vi "Test Ultrasonic Sensor VI.vi"() -> ()   [LabVIEW 2017]
uses:
  <vilib>/Rock Robotics/SystemInterfaces/AI/FPGA_AIChannel.ctl
  <vilib>/Rock Robotics/WPI/Ultrasonic/WPI_SonarMB1010AnalogOpen.vi
  <vilib>/Rock Robotics/WPI/Ultrasonic/WPI_SonarMB1010AnalogRefNum Registry Set.vi
  <vilib>/Rock Robotics/WPI/Ultrasonic/WPI_SonarMB1010AnalogRefNum Registry Get.vi
panel:
  out "Distance":dbl
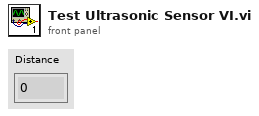
[diagram p1: front panel]
types:
  T1 = typedef "FPGA_AIChannel.ctl" = enum8{"AI 0", "AI 1", "AI 2", "AI 3", "AI MXP 0", "AI MXP 1", "AI MXP 2", "AI MXP 3", "Invalid"}
  T2 = typedef "WPI_SonarMB1010AnalogDeviceRef.ctl" = cluster{"AIDeviceRef":T3, "Scaling factor (V/in)":dbl, "Average Bits":u8}
  T3 = typedef "WPI_AnalogChannelDevRef.ctl" = cluster{"DevStatus":errorcluster, "Analog Channel":T1}
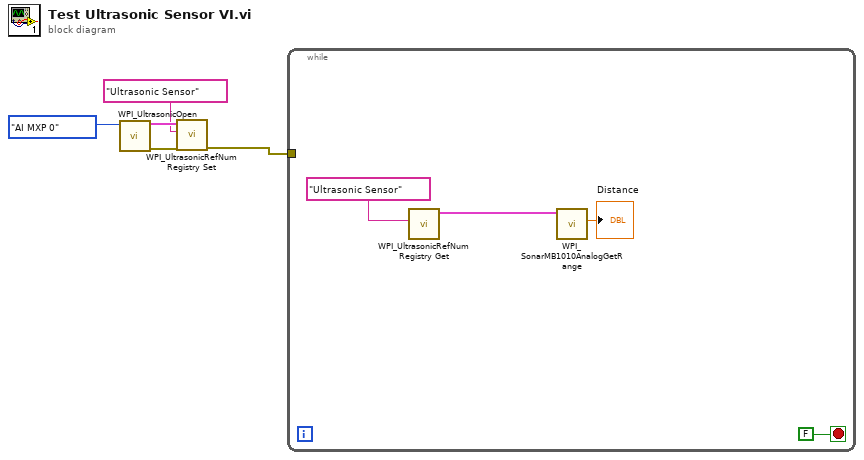
[diagram p0: block diagram]
diagram:
  n1 = call-poly <vilib>:"WPI_UltrasonicOpen.vi"("Analog Channel"=FPGA_AIChannel."AI MXP 0") -> ("error out"=w5:errorcluster, "SonarMB1010AnalogDevRef"=w4:T2)  [unwired: 9 in]
  n2 = call-poly <vilib>:"WPI_UltrasonicRefNum Registry Set.vi"("error in (no error)"=w5, "refnum name"="Ultrasonic Sensor", "SonarMB1010AnalogDevRef"=w4) -> ("error out"=w1:errorcluster)  [unwired: 7 in, 1 out]
  n3 = while {
    tunnel: w1 -> [_]
    stop <- FALSE stop-if-true
    n4 = call-poly <vilib>:"WPI_UltrasonicRefNum Registry Get.vi"("refnum name"="Ultrasonic Sensor") -> ("SonarMB1010AnalogDevRef"=w7:T2)  [unwired: 9 in, 1 out]
    n5 = call <vilib>:"WPI_SonarMB1010AnalogGetRange.vi"("SonarMB1010AnalogDevRef"=w7) -> ("Distance"=→"Distance":dbl)  [unwired: 8 in, 2 out]
  }
